vi "Change Motor High Time.vi"(8 "error in":errorcluster, 11 "tCRD in":refnum<class "Aircraft OPCCRD.lvclass">) -> (0 "error out":errorcluster, 3 "tCRD out":refnum<class "Aircraft OPCCRD.lvclass">)   [LabVIEW 2015, in "Aircraft OPCCRD.lvclass"]
doc: "This controls the PWM signal on the servo which is used to open and close the sample line. Most servos operate on a 50 Hz PWM signal, with high times varying between 1-2 ms. Some motors do have endpoints at lower and higher times, but this is a general configuration."
uses:
  Aircraft OPCCRD.lvclass
  tFPGA Ref.ctl
  <vilib>/rvi/interface/nirviReadWriteControl/nirviReadWriteControl.xnode
  Reusable/Instrument/Instrument.lvclass
  Reusable/CRDS/Data/Main/CRDS Data.lvclass
  Switch/Servo Switch.lvclass
  FPGA Bitfiles/FPGAServerwLRS.lvbitx
  NiFpgaLv.dll
  <vilib>/Utility/error.llb/Error Cluster From Error Code.vi
  <vilib>/rvi/errors/niLvFpgaAdjustHostInterfaceError.vi
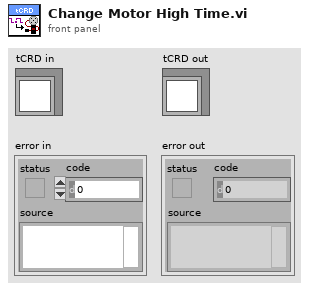
[diagram p1: front panel]
types:
  T1 = typedef "Aircraft OPCCRD.lvclass/tFPGA Ref.ctl" = refnum<k20>
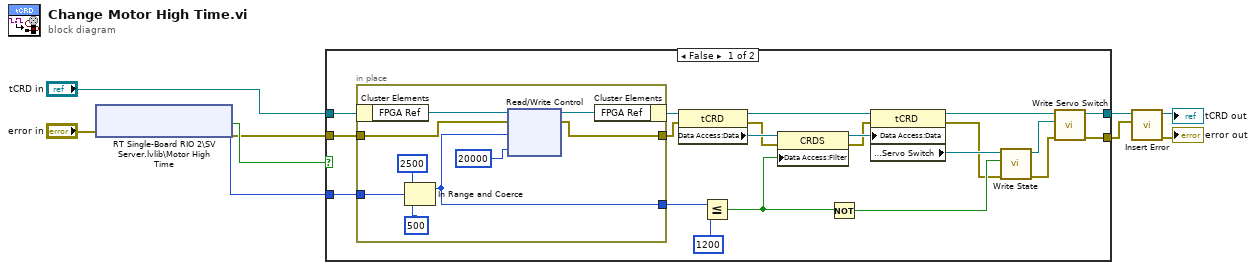
[diagram p0: block diagram]
diagram:
  n1 = shared-variable "RT Single-Board RIO 2\\SV Server.lvlib\\Motor High Time"(error in="error in") -> (w8:u32, error out=w7:errorcluster, w9:bool)  [unwired: 1 in]
  n2 = case shown="False" w9 {
    tunnel: "tCRD in" -> [w29 w41]
    tunnel: [w13 w41] -> w4
    tunnel: w8 -> [w30 _]
    tunnel: w7 -> [w28 w40]
    tunnel: [w12 w40] -> w3
    frame False {
      n3 = in-place {
        in-place-border: w30 -> [w35]
        in-place-border: w28 -> [w37]
        in-place-border: [w36] -> w26
        in-place-border: [w31] -> w19
        n4 = in-place-cluster #1(w29) -> ("FPGA Ref"=w39:T1)
        n5 = In Range and Coerce(upper limit=u32 2500, x=w35, lower limit=u32 500) -> (coerced(x)=w31:u32)  [unwired: 1 out]
        n6 = xnode "Read/Write Control"("FPGA VI Reference In"=w39, "error in"=w37, "High"=w31, "Low"=u32 20000 ("x")) -> ("FPGA VI Reference Out"=w38:T1, "error out"=w36:errorcluster)
        n7 = in-place-cluster #1("FPGA Ref"=w38) -> (w27:refnum<class "Aircraft OPCCRD.lvclass">)
      }
      n8 = property class="tCRD"(reference=w27, error in=w26) -> (reference out=w25:refnum<class "Aircraft OPCCRD.lvclass">, error out=w21:errorcluster, "Data Access:Data"=w24:refnum<class "CRDS Data.lvclass">)
      n9 = Less Or Equal?(x=w19, y=u32 1200) -> (x <= y?=w18:bool)
      n10 = property class="CRDS"(reference=w24, error in=w21, "Data Access:Filter"=w18) -> (reference out=w23:refnum<class "CRDS Data.lvclass">, error out=w22:errorcluster)
      n11 = Not(x=w18) -> (.not. x?=w16:bool)
      n12 = property class="tCRD"(reference=w25, error in=w22, "Data Access:Data"=w23) -> (reference out=w14:refnum<class "Aircraft OPCCRD.lvclass">, error out=w15:errorcluster, "Accessors:Servo Switch"=w17:refnum<class "Servo Switch.lvclass">)
      n13 = call-dynamic "Write State.vi"("error in"=w15, "State"=w16, "Switch in"=w17) -> ("error out"=w11:errorcluster, "Switch out"=w10:refnum<class "Servo Switch.lvclass">)  [unwired: 7 in]
      n14 = call "Write Servo Switch.vi"("error in (no error)"=w11, "Servo Switch"=w10, "tCRD in"=w14) -> ("error out"=w12:errorcluster, "tCRD out"=w13:refnum<class "Aircraft OPCCRD.lvclass">)  [unwired: 7 in]
    }
    frame True {
    }
  }
  n15 = call "Insert Error.vi"("err"=w3, "Instrument in"=w4) -> ("error out"=→"error out":errorcluster, "Instrument out"=→"tCRD out":refnum<class "Aircraft OPCCRD.lvclass">)  [unwired: 7 in, 1 out]
